vi "Init DB.vi"(8 "error in (no error)":errorcluster, 11 "UserPwd DB in":refnum<class "UserPwd DB.lvclass">) -> (0 "error out":errorcluster, 3 "UserPwd DB out":refnum<class "UserPwd DB.lvclass">)   [LabVIEW 2016, in "UserPwd DB.lvlib" / "UserPwd DB.lvclass"]
uses:
  <userlib>/Common Components/UserPwd DB/UserPwd DB/UserPwd DB.lvclass
  <userlib>/Common Components/UserPwd DB/UserPwd DB/Data saved.ctl
  <userlib>/Common Components/UserPwd DB/UserPwd DB/Access Level.ctl
  <userlib>/Common Components/UserPwd DB/UserPwd DB/UserPwd DB.lvclass/UserPwd DB.ctl
  <vilib>/addons/_JKI.lib/Serialization/JSON/JKI JSON Serialization.lvlib
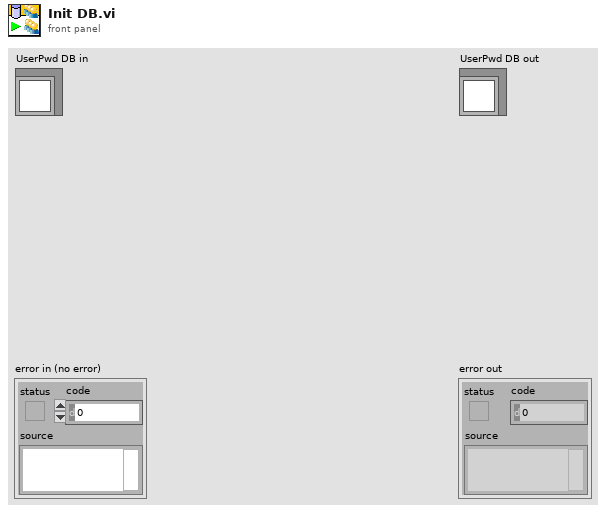
[diagram p1: front panel]
types:
  T1 = typedef "UserPwd DB.lvlib/UserPwd DB.lvclass/Data saved.ctl" = cluster{"Encrypted Password":string, "Access":T2, "Permission":u32}
  T2 = typedef "UserPwd DB.lvlib/UserPwd DB.lvclass/Access Level.ctl" = enum16{"Admin", "User lv1", "User lv2", "User lv3", "User lv4", "User lv5", "User lv6", "User lv7", "User lv8", "User lv9", "Guest"}
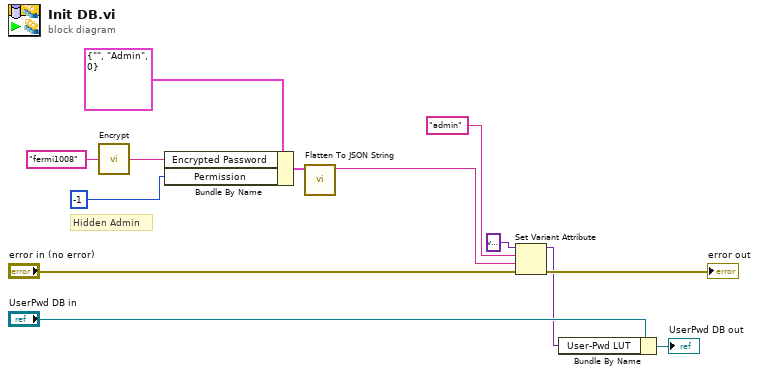
[diagram p0: block diagram]
diagram:
  # "Hidden Admin"
  n1 = call <userlib>:"Encrypt.vi"("String"="fermi1008") -> ("Encrypted String"=w5:string)
  n2 = Bundle By Name(cluster=T1 {"Encrypted Password"="", "Access"=enum."Admin", "Permission"=0} ("Data"), "Encrypted Password"=w5, "Permission"=-1) -> (w4:T1)
  n3 = call <vilib>:"Flatten To JSON String.vi"("Variant"=w4) -> ("JSON String"=w2:string)  [unwired: 9 in, 1 out]
  n4 = Set Variant Attribute(Variant=variant ("variant"), name="admin", value=w2, error in="error in (no error)") -> (Variant out=w3:variant, error out=→"error out":errorcluster)  [unwired: 1 out]
  n5 = Bundle By Name(cluster="UserPwd DB in", "User-Pwd LUT"=w3) -> (→"UserPwd DB out":refnum<class "UserPwd DB.lvclass">)
